vi "LoginOPCDL.vi"() -> (2 "output cluster":cluster{"Username":string, "Password":string})   [LabVIEW 2025]
panel:
  in  "OK Button":bool
  in  "Password":string
  in  "Username":string
  # "Login OPC Server"
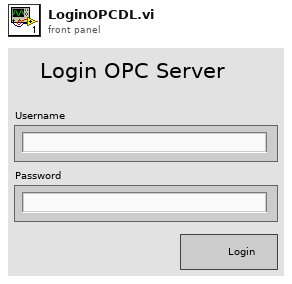
[diagram p1: front panel]
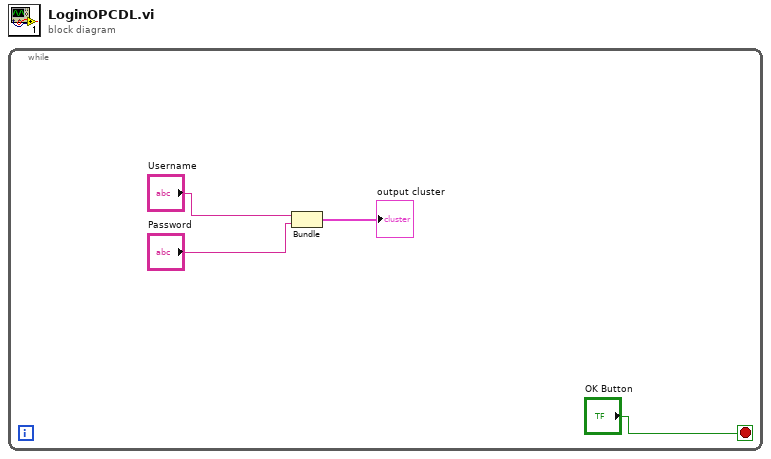
[diagram p0: block diagram]
diagram:
  n1 = while {
    stop <- "OK Button" stop-if-true
    n2 = Bundle("Username"="Username", "Password"="Password") -> (→"output cluster":cluster{"Username":string, "Password":string})  [unwired: 1 in]
  }
